vi "LWXPS_ZygoInterferometerStatusGet.vi"(0 "XPS Reference IN":refnum<k24>, 11 "LabVIEW error IN":errorcluster) -> (2 "XPS Reference OUT":refnum<k24>, 3 "Returned error code":i32, 4 "Ethernet communication status":i32, 6 "Zygo axis 1 measure signal":i32, 8 "Zygo axis 2 measure signal":i32, 10 "Zygo reference signal status":i32, 13 "LabVIEW error OUT":errorcluster, 14 "XPS Error String":string, 15 "Zygo P2 board status":i32)   [LabVIEW 2014]
uses:
  D:/XPSQ8_LabView_Library/Development/Source/Dll/Newport.XPS.CommandInterface.dll
  Dll/Newport.XPS.CommandInterface.dll
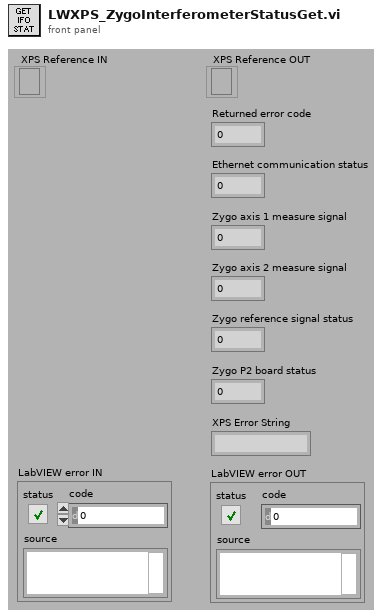
[diagram p1: front panel]
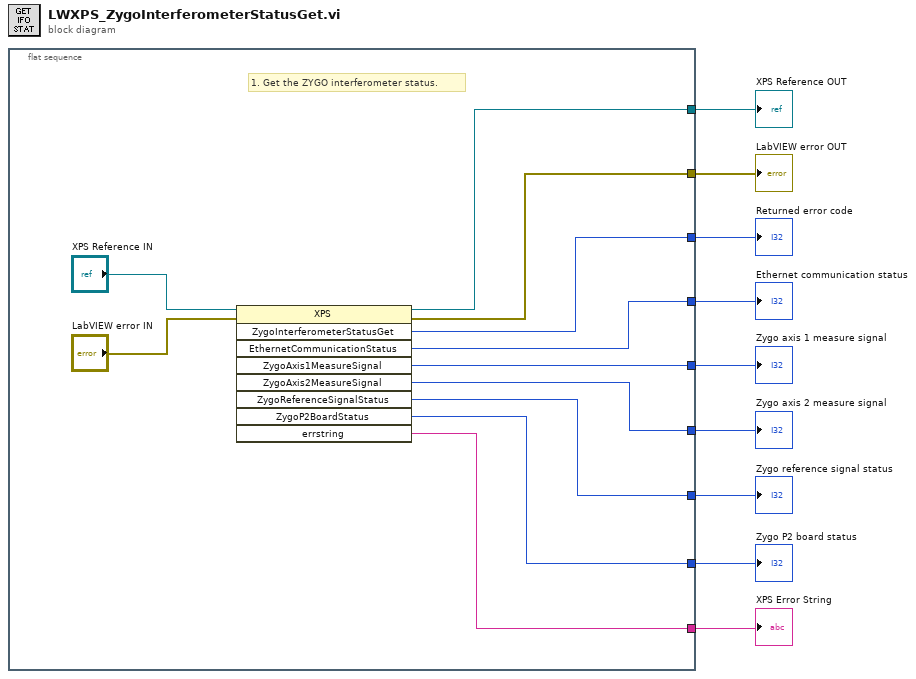
[diagram p0: block diagram]
diagram:
  n1 = flat-sequence {
    tunnel: [w18] -> w9
    tunnel: [w16] -> w8
    tunnel: [w19] -> w7
    tunnel: [w14] -> w6
    tunnel: [w15] -> w5
    tunnel: [w13] -> w1
    tunnel: [w12] -> w2
    tunnel: [w11] -> w4
    tunnel: [w10] -> w3
    frame #0 {
      # "1. Get the ZYGO interferometer status."
      n2 = invoke class="XPS" method="ZygoInterferometerStatusGet"(reference="XPS Reference IN", error in="LabVIEW error IN") -> (reference out=w18:refnum<k24>, error out=w16:errorcluster, "ZygoInterferometerStatusGet"=w19:i32, "EthernetCommunicationStatus"=w11:i32, "ZygoAxis1MeasureSignal"=w14:i32, "ZygoAxis2MeasureSignal"=w15:i32, "ZygoReferenceSignalStatus"=w13:i32, "ZygoP2BoardStatus"=w12:i32, "errstring"=w10:string)  [unwired: 7 in]
    }
  }
  "XPS Error String" <- w3
  "XPS Reference OUT" <- w9
  "LabVIEW error OUT" <- w8
  "Returned error code" <- w7
  "Zygo axis 1 measure signal" <- w6
  "Zygo axis 2 measure signal" <- w5
  "Ethernet communication status" <- w4
  "Zygo P2 board status" <- w2
  "Zygo reference signal status" <- w1
